vi "Write X.vi"(8 "error in (no error)":errorcluster, 10 "X":dbl[][](array[numeric]), 11 "StateFunction in":refnum<class "StateFunction.lvclass">) -> (0 "error out":errorcluster, 3 "StateFunction out":refnum<class "StateFunction.lvclass">)   [LabVIEW 2014, in "StateFunction.lvclass"]
uses:
  StateFunction.lvclass
  StateFunction.lvclass/StateFunction.ctl
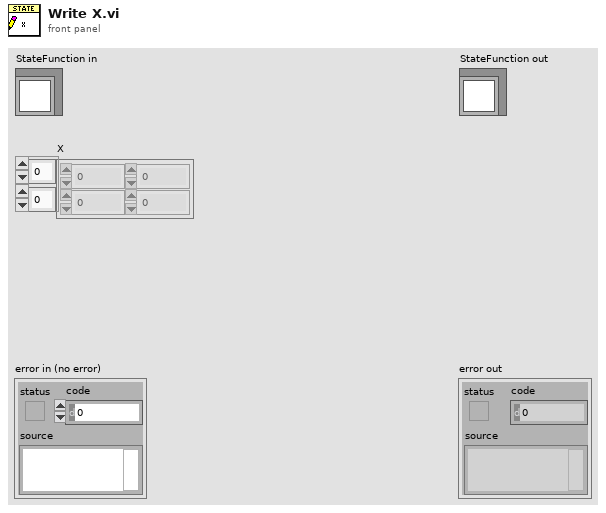
[diagram p1: front panel]
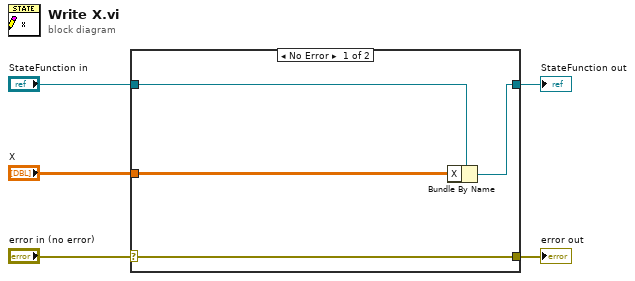
[diagram p0: block diagram]
diagram:
  n1 = case shown="No Error" "error in (no error)" {
    selector: "error in (no error)" -> [w9 w10]
    tunnel: [w9 w10] -> w4
    tunnel: [w7 w11] -> w2
    tunnel: "StateFunction in" -> [w8 w11]
    tunnel: "X" -> [w6 _]
    frame No Error {
      n2 = Bundle By Name(cluster=w8, "X"=w6) -> (w7:refnum<class "StateFunction.lvclass">)
    }
    frame Error {
    }
  }
  "error out" <- w4
  "StateFunction out" <- w2
